vi "KubelkaMunk.vi"(1 "Reflectance":dbl) -> (0 "K/S":dbl)   [LabVIEW 2013]
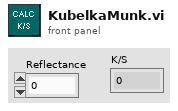
[diagram p1: front panel]
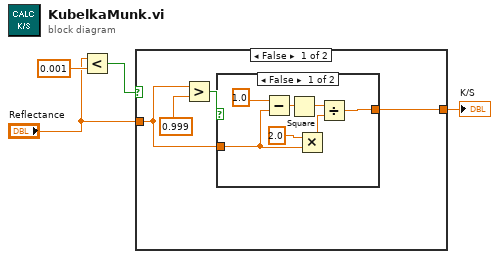
[diagram p0: block diagram]
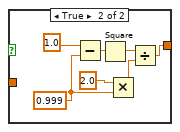
[diagram p2: hidden frame]
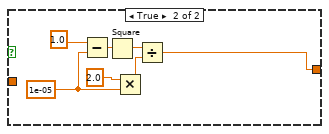
[diagram p3: hidden frame]
diagram:
  n1 = Less?(x="Reflectance", y=0.001) -> (x < y?=w3:bool)
  n2 = case shown="False" w3 {
    tunnel: [w8 w24] -> w1
    tunnel: "Reflectance" -> [w7 _]
    frame False {
      n3 = Greater?(x=w7, y=0.999) -> (0:w5:bool)
      n4 = case shown="False" w5 {
        tunnel: [w9 w17] -> w8
        tunnel: w7 -> [w10 _]
        frame False {
          n5 = Subtract(x=1.0, y=w10) -> (x-y=w14:dbl)
          n6 = Square(x=w14) -> (x^2=w12:dbl)
          n7 = Multiply(x=2.0, y=w10) -> (x*y=w11:dbl)
          n8 = Divide(x=w12, y=w11) -> (x/y=w9:dbl)
        }
        frame True {
          w16 = 0.999 ("y")
          n9 = Subtract(x=1.0, y=w16) -> (x-y=w21:dbl)
          n10 = Square(x=w21) -> (x^2=w19:dbl)
          n11 = Multiply(x=2.0, y=w16) -> (x*y=w18:dbl)
          n12 = Divide(x=w19, y=w18) -> (x/y=w17:dbl)
        }
      }
    }
    frame True {
      w23 = 1e-05 ("y")
      n13 = Subtract(x=1.0, y=w23) -> (x-y=w28:dbl)
      n14 = Square(x=w28) -> (x^2=w26:dbl)
      n15 = Multiply(x=2.0, y=w23) -> (x*y=w25:dbl)
      n16 = Divide(x=w26, y=w25) -> (x/y=w24:dbl)
    }
  }
  "K/S" <- w1
